vi "ServoTest.vi"(10 "Down":bool=TRUE, 11 "Up":bool=TRUE) -> (3 "Angle":dbl)   [LabVIEW 2018]
panel:
  in  "Rate":dbl format="%#_13g"
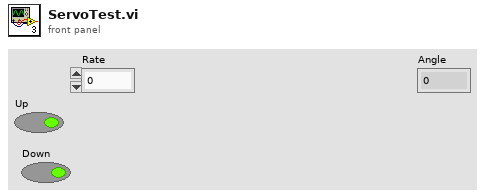
[diagram p1: front panel]
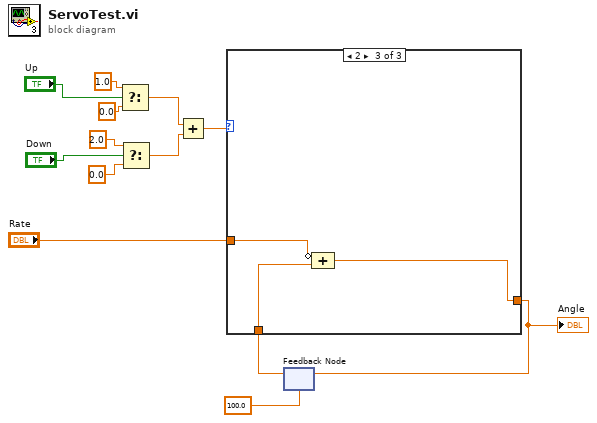
[diagram p0: block diagram]
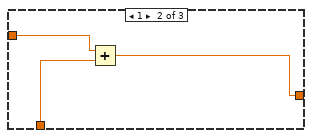
[diagram p3: hidden frame]
diagram:
  n1 = Select(t=1.0, s="Up", f=0.0) -> (s? t:f=w7:dbl)
  n2 = Select(t=2.0, s="Down", f=0.0) -> (s? t:f=w6:dbl)
  n3 = Add(x=w7, y=w6) -> (x+y=w5:dbl)
  n4 = feedback #1(100.0 ("f")) -> (w3:dbl)
  n5 = case shown="2" w5 {
    tunnel: w3 -> [w14 w17 w20]
    tunnel: [w14 w16 w19] -> w2
    tunnel: "Rate" -> [_ w15 w18]
    frame 0, Default {
    }
    frame 1 {
      n6 = Add(x=w15, y=w17) -> (x+y=w16:dbl)
    }
    frame 2 {
      n7 = Compound Arithmetic op=ADD(invert w18, w20) -> (w19:dbl)
    }
  }
  "Angle" <- w2
  n8 = feedback-in #1(w2) -> ()
